vi "测试类型1can请求.vi"(3 "输入切换ID":u8, 4 "输出切换ID":u8) -> (1 "发送成功?":bool)   [LabVIEW 2010]
panel:
  in  "DataLen":i16
  in  "Data":u8[](array[numeric])
  in  "CANPort":u16
  in  "Synchronization":i32(ring)=1 items=["Synchronization"=1, "Asynchronization"=0]
  in  "WriteTimeOut":u32=5000 caption="ms"
  in  "Baudrate":u32(ring)=1000 caption="K" items=["10"=10, "20"=20, "50"=50, "100"=100, "125"=125, "250"=250, "500"=500, "800"=800, "1000"=1000]
  in  "Send_MSG":T1(array[cluster])=[{"Flags"=4, "ID(HEX)"=0, "Data "=[0, 0, 0, 0, 0, 0, 0, 0]}, {"Flags"=4, "ID(HEX)"=0, "Data "=[0, 0, 0, 0, 0, 0, 0, 1]}, {"Flags"=4, "ID(HEX)"=0, "Data "=[0, 0, 0, 0, 0, 0, 0, 2]}, {"Flags"=4, "ID(HEX)"=0, "Data "=[0, 0, 0, 0, 0, 0, 0, 3]}, {"Flags"=4, "ID(HEX)"=0, "Data "=[0, 0, 0, 0, 0, 0, 0, 4]}, {"Flags"=4, "ID(HEX)"=0, "Data "=[0, 0, 0, 0, 0, 0, 0, 5]}, {"Flags"=4, "ID(HEX)"=0, "Data "=[0, 0, 0, 0, 0, 0, 0, 6]}, {"Flags"=4, "ID(HEX)"=0, "Data "=[0, 0, 0, 0, 0, 0, 0, 7]}, {"Flags"=4, "ID(HEX)"=0, "Data "=[0, 0, 0, 0, 0, 0, 0, 8]}, {"Flags"=4, "ID(HEX)"=0, "Data "=[0, 0, 0, 0, 0, 0, 0, 9]}, {"Flags"=4, "ID(HEX)"=0, "Data "=[0, 0, 0, 0, 0, 0, 1, 0]}, {"Flags"=4, "ID(HEX)"=0, "Data "=[0, 0, 0, 0, 0, 0, 1, 1]}, {"Flags"=4, "ID(HEX)"=0, "Data "=[0, 0, 0, 0, 0, 0, 1, 2]}, {"Flags"=4, "ID(HEX)"=0, "Data "=[0, 0, 0, 0, 0, 0, 1, 3]}, {"Flags"=4, "ID(HEX)"=0, "Data "=[0, 0, 0, 0, 0, 0, 1, 4]}, {"Flags"=4, "ID(HEX)"=0, "Data "=[0, 0, 0, 0, 0, 0, 1, 5]}, {"Flags"=4, "ID(HEX)"=0, "Data "=[0, 0, 0, 0, 0, 0, 1, 6]}, {"Flags"=4, "ID(HEX)"=0, "Data "=[0, 0, 0, 0, 0, 0, 1, 7]}, {"Flags"=4, "ID(HEX)"=0, "Data "=[0, 0, 0, 0, 0, 0, 1, 8]}, {"Flags"=4, "ID(HEX)"=0, "Data "=[0, 0, 0, 0, 0, 0, 1, 9]}, {"Flags"=4, "ID(HEX)"=0, "Data "=[0, 0, 0, 0, 0, 0, 2, 0]}, {"Flags"=4, "ID(HEX)"=0, "Data "=[0, 0, 0, 0, 0, 0, 2, 1]}, {"Flags"=4, "ID(HEX)"=0, "Data "=[0, 0, 0, 0, 0, 0, 2, 2]}, {"Flags"=4, "ID(HEX)"=0, "Data "=[0, 0, 0, 0, 0, 0, 2, 3]}, {"Flags"=4, "ID(HEX)"=0, "Data "=[0, 0, 0, 0, 0, 0, 2, 4]}, {"Flags"=4, "ID(HEX)"=0, "Data "=[0, 0, 0, 0, 0, 0, 2, 5]}, {"Flags"=4, "ID(HEX)"=0, "Data "=[0, 0, 0, 0, 0, 0, 2, 6]}, {"Flags"=4, "ID(HEX)"=0, "Data "=[0, 0, 0, 0, 0, 0, 2, 7]}, {"Flags"=4, "ID(HEX)"=0, "Data "=[0, 0, 0, 0, 0, 0, 2, 8]}, {"Flags"=4, "ID(HEX)"=0, "Data "=[0, 0, 0, 0, 0, 0, 2, 9]}, {"Flags"=4, "ID(HEX)"=0, "Data "=[0, 0, 0, 0, 0, 0, 3, 0]}, {"Flags"=4, "ID(HEX)"=0, "Data "=[0, 0, 0, 0, 0, 0, 3, 1]}, {"Flags"=4, "ID(HEX)"=0, "Data "=[0, 0, 0, 0, 0, 0, 3, 2]}, {"Flags"=4, "ID(HEX)"=0, "Data "=[0, 0, 0, 0, 0, 0, 3, 3]}, {"Flags"=4, "ID(HEX)"=0, "Data "=[0, 0, 0, 0, 0, 0, 3, 4]}, {"Flags"=4, "ID(HEX)"=0, "Data "=[0, 0, 0, 0, 0, 0, 3, 5]}, {"Flags"=4, "ID(HEX)"=0, "Data "=[0, 0, 0, 0, 0, 0, 3, 6]}, {"Flags"=4, "ID(HEX)"=0, "Data "=[0, 0, 0, 0, 0, 0, 3, 7]}, {"Flags"=4, "ID(HEX)"=0, "Data "=[0, 0, 0, 0, 0, 0, 3, 8]}, {"Flags"=4, "ID(HEX)"=0, "Data "=[0, 0, 0, 0, 0, 0, 3, 9]}, {"Flags"=4, "ID(HEX)"=0, "Data "=[0, 0, 0, 0, 0, 0, 4, 0]}, {"Flags"=4, "ID(HEX)"=0, "Data "=[0, 0, 0, 0, 0, 0, 4, 1]}, {"Flags"=4, "ID(HEX)"=0, "Data "=[0, 0, 0, 0, 0, 0, 4, 2]}, {"Flags"=4, "ID(HEX)"=0, "Data "=[0, 0, 0, 0, 0, 0, 4, 3]}, {"Flags"=4, "ID(HEX)"=0, "Data "=[0, 0, 0, 0, 0, 0, 4, 4]}, {"Flags"=4, "ID(HEX)"=0, "Data "=[0, 0, 0, 0, 0, 0, 4, 5]}, {"Flags"=4, "ID(HEX)"=0, "Data "=[0, 0, 0, 0, 0, 0, 4, 6]}, {"Flags"=4, "ID(HEX)"=0, "Data "=[0, 0, 0, 0, 0, 0, 4, 7]}, {"Flags"=4, "ID(HEX)"=0, "Data "=[0, 0, 0, 0, 0, 0, 4, 8]}, {"Flags"=4, "ID(HEX)"=0, "Data "=[0, 0, 0, 0, 0, 0, 4, 9]}, {"Flags"=4, "ID(HEX)"=0, "Data "=[0, 0, 0, 0, 0, 0, 5, 0]}, {"Flags"=4, "ID(HEX)"=0, "Data "=[0, 0, 0, 0, 0, 0, 5, 1]}, {"Flags"=4, "ID(HEX)"=0, "Data "=[0, 0, 0, 0, 0, 0, 5, 2]}, {"Flags"=4, "ID(HEX)"=0, "Data "=[0, 0, 0, 0, 0, 0, 5, 3]}, {"Flags"=4, "ID(HEX)"=0, "Data "=[0, 0, 0, 0, 0, 0, 5, 4]}, {"Flags"=4, "ID(HEX)"=0, "Data "=[0, 0, 0, 0, 0, 0, 5, 5]}, {"Flags"=4, "ID(HEX)"=0, "Data "=[0, 0, 0, 0, 0, 0, 5, 6]}, {"Flags"=4, "ID(HEX)"=0, "Data "=[0, 0, 0, 0, 0, 0, 5, 7]}, {"Flags"=4, "ID(HEX)"=0, "Data "=[0, 0, 0, 0, 0, 0, 5, 8]}, {"Flags"=4, "ID(HEX)"=0, "Data "=[0, 0, 0, 0, 0, 0, 5, 9]}, {"Flags"=4, "ID(HEX)"=0, "Data "=[0, 0, 0, 0, 0, 0, 6, 0]}, {"Flags"=4, "ID(HEX)"=0, "Data "=[0, 0, 0, 0, 0, 0, 6, 1]}, {"Flags"=4, "ID(HEX)"=0, "Data "=[0, 0, 0, 0, 0, 0, 6, 2]}, {"Flags"=4, "ID(HEX)"=0, "Data "=[0, 0, 0, 0, 0, 0, 6, 3]}, {"Flags"=4, "ID(HEX)"=0, "Data "=[0, 0, 0, 0, 0, 0, 6, 4]}, {"Flags"=4, "ID(HEX)"=0, "Data "=[0, 0, 0, 0, 0, 0, 6, 5]}, {"Flags"=4, "ID(HEX)"=0, "Data "=[0, 0, 0, 0, 0, 0, 6, 6]}, {"Flags"=4, "ID(HEX)"=0, "Data "=[0, 0, 0, 0, 0, 0, 6, 7]}, {"Flags"=4, "ID(HEX)"=0, "Data "=[0, 0, 0, 0, 0, 0, 6, 8]}, {"Flags"=4, "ID(HEX)"=0, "Data "=[0, 0, 0, 0, 0, 0, 6, 9]}, {"Flags"=4, "ID(HEX)"=0, "Data "=[0, 0, 0, 0, 0, 0, 7, 0]}, {"Flags"=4, "ID(HEX)"=0, "Data "=[0, 0, 0, 0, 0, 0, 7, 1]}, {"Flags"=4, "ID(HEX)"=0, "Data "=[0, 0, 0, 0, 0, 0, 7, 2]}, {"Flags"=4, "ID(HEX)"=0, "Data "=[0, 0, 0, 0, 0, 0, 7, 3]}, {"Flags"=4, "ID(HEX)"=0, "Data "=[0, 0, 0, 0, 0, 0, 7, 4]}, {"Flags"=4, "ID(HEX)"=0, "Data "=[0, 0, 0, 0, 0, 0, 7, 5]}, {"Flags"=4, "ID(HEX)"=0, "Data "=[0, 0, 0, 0, 0, 0, 7, 6]}, {"Flags"=4, "ID(HEX)"=0, "Data "=[0, 0, 0, 0, 0, 0, 7, 7]}, {"Flags"=4, "ID(HEX)"=0, "Data "=[0, 0, 0, 0, 0, 0, 7, 8]}, {"Flags"=4, "ID(HEX)"=0, "Data "=[0, 0, 0, 0, 0, 0, 7, 9]}, {"Flags"=4, "ID(HEX)"=0, "Data "=[0, 0, 0, 0, 0, 0, 8, 0]}, {"Flags"=4, "ID(HEX)"=0, "Data "=[0, 0, 0, 0, 0, 0, 8, 1]}, {"Flags"=4, "ID(HEX)"=0, "Data "=[0, 0, 0, 0, 0, 0, 8, 2]}, {"Flags"=4, "ID(HEX)"=0, "Data "=[0, 0, 0, 0, 0, 0, 8, 3]}, {"Flags"=4, "ID(HEX)"=0, "Data "=[0, 0, 0, 0, 0, 0, 8, 4]}, {"Flags"=4, "ID(HEX)"=0, "Data "=[0, 0, 0, 0, 0, 0, 8, 5]}, {"Flags"=4, "ID(HEX)"=0, "Data "=[0, 0, 0, 0, 0, 0, 8, 6]}, {"Flags"=4, "ID(HEX)"=0, "Data "=[0, 0, 0, 0, 0, 0, 8, 7]}, {"Flags"=4, "ID(HEX)"=0, "Data "=[0, 0, 0, 0, 0, 0, 8, 8]}, {"Flags"=4, "ID(HEX)"=0, "Data "=[0, 0, 0, 0, 0, 0, 8, 9]}, {"Flags"=4, "ID(HEX)"=0, "Data "=[0, 0, 0, 0, 0, 0, 9, 0]}, {"Flags"=4, "ID(HEX)"=0, "Data "=[0, 0, 0, 0, 0, 0, 9, 1]}, {"Flags"=4, "ID(HEX)"=0, "Data "=[0, 0, 0, 0, 0, 0, 9, 2]}, {"Flags"=4, "ID(HEX)"=0, "Data "=[0, 0, 0, 0, 0, 0, 9, 3]}, {"Flags"=4, "ID(HEX)"=0, "Data "=[0, 0, 0, 0, 0, 0, 9, 4]}, {"Flags"=4, "ID(HEX)"=0, "Data "=[0, 0, 0, 0, 0, 0, 9, 5]}, {"Flags"=4, "ID(HEX)"=0, "Data "=[0, 0, 0, 0, 0, 0, 9, 6]}, {"Flags"=4, "ID(HEX)"=0, "Data "=[0, 0, 0, 0, 0, 0, 9, 7]}, {"Flags"=4, "ID(HEX)"=0, "Data "=[0, 0, 0, 0, 0, 0, 9, 8]}, {"Flags"=4, "ID(HEX)"=0, "Data "=[0, 0, 0, 0, 0, 0, 9, 9]}] {"Data" format="%x"; "Flags" items=["MSG_STD"=0, "MSG_EXT"=4]; "ID(HEX)" format="%x"}
  out "Error out":errorcluster {"code" format="%.0x"}
  in  "CANID":u32 format="%x"
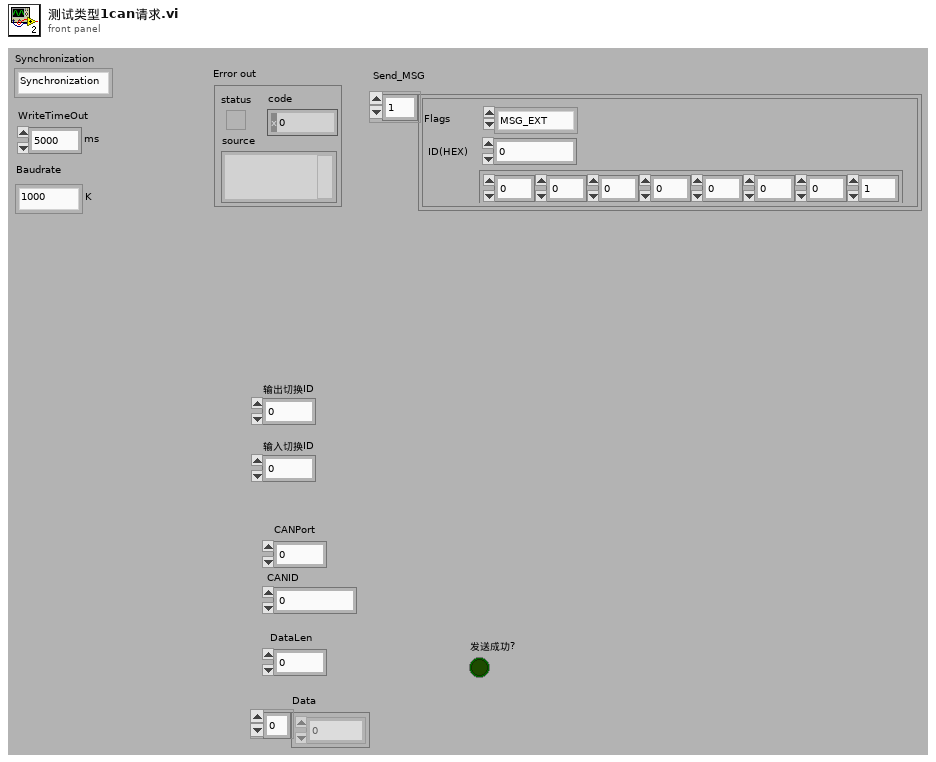
[diagram p1: front panel]
types:
  T1 = cluster{"Flags":u32, "ID(HEX)":u32, "Data ":u8[]}[]
  T2 = cluster{"Internal":u32, "InternalHigh":u32, "Offset":u32, "OffsetHigh":u32, "hEvent":u32}
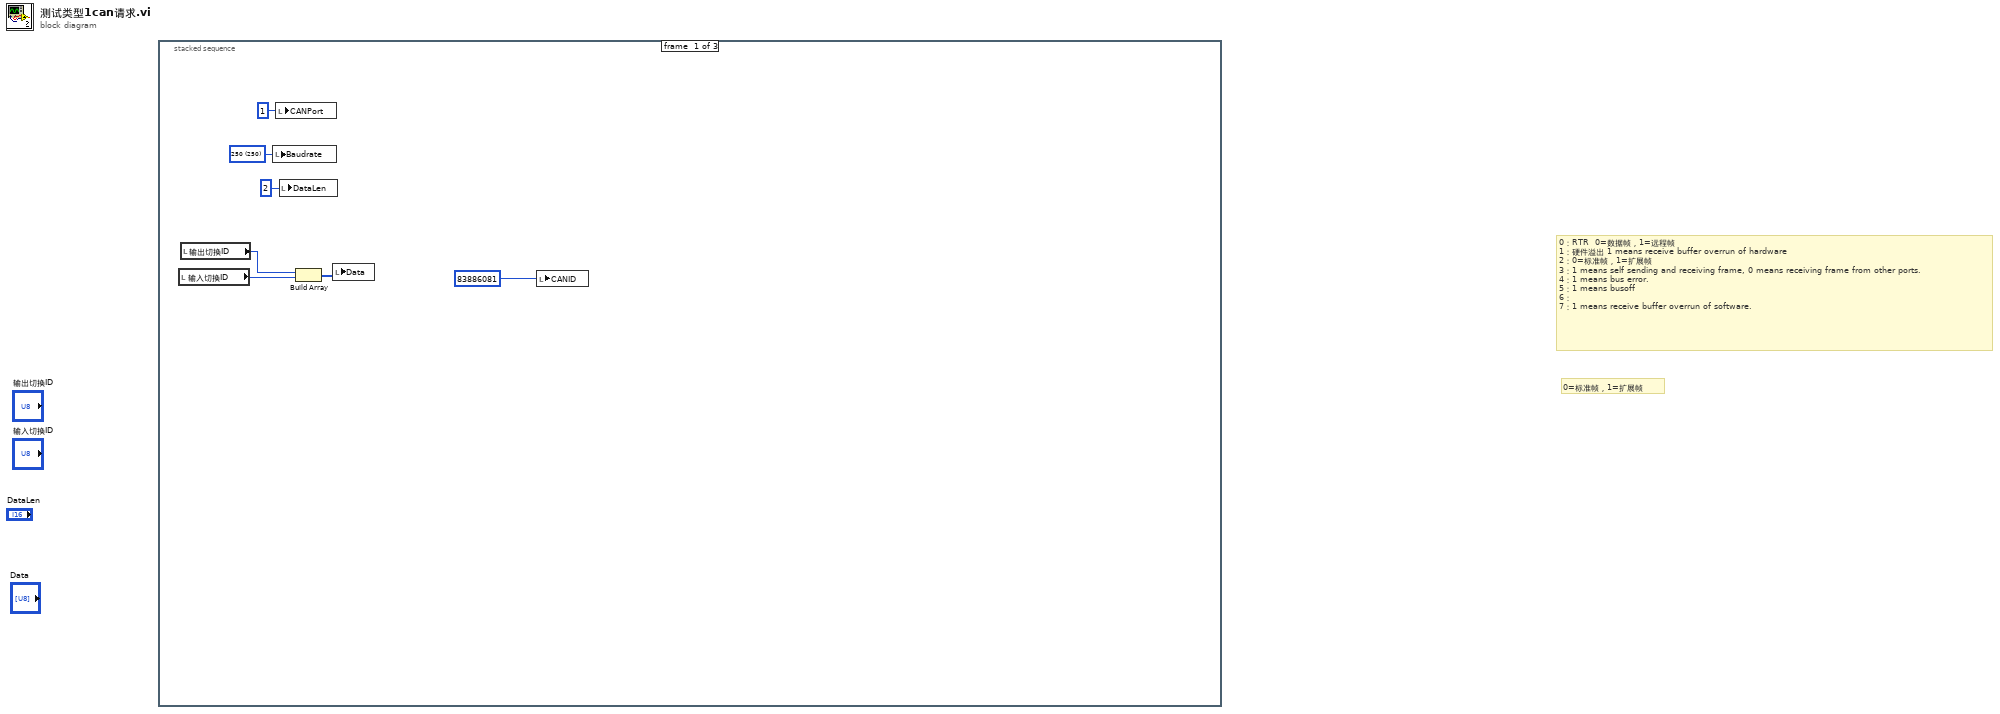
[diagram p0: block diagram]
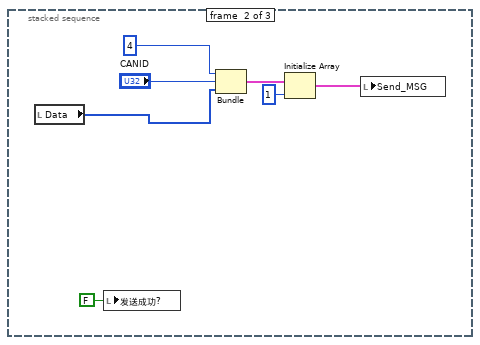
[diagram p2: hidden frame]
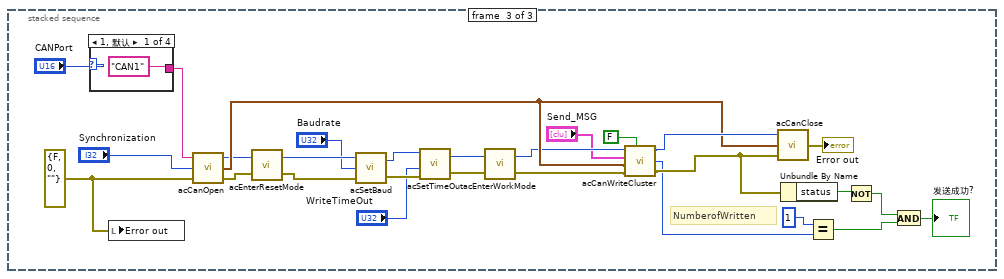
[diagram p3: hidden frame]
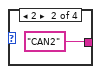
[diagram p4: hidden frame]
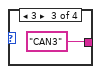
[diagram p5: hidden frame]
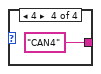
[diagram p6: hidden frame]
diagram:
  # "0=标准帧，1=扩展帧"
  # "0：RTR  0=数据帧，1=远程帧\n1：硬件溢出 1 means receive buffer overrun of hardware\n2：0=标准帧，1=扩展帧\n3：1 means self sending and receiving frame, 0 means receiving frame from other ports.\n4：1 means bus error.\n5：1 means busoff\n6：\n7：1 means receive buffer overrun of software."
  n1 = stacked-sequence {
    frame #0 {
      w7 = u32 250 items=["10"=10, "20"=20, "50"=50, "100"=100, "125"=125, "250"=250, "500"=500, "800"=800, "1000"=1000] ("Baudrate")
      n2 = local read "输入切换ID"() -> (w2:u8)
      n3 = local read "输出切换ID"() -> (w3:u8)
      n4 = local write "Baudrate"(w7) -> ()
      n5 = local write "CANPort"(u16 1 ("CANPort")) -> ()
      n6 = local write "DataLen"(i16 2 ("DataLen")) -> ()
      n7 = Build Array(w3, w2) -> (w4:u8[])
      n8 = local write "Data"(w4) -> ()
      n9 = local write "CANID"(u32 83886081 ("CANID")) -> ()
    }
    frame #1 {
      n10 = local read "Data"() -> (w8:u8[])
      n11 = local write "发送成功?"(FALSE ("发送成功?")) -> ()
      n12 = Bundle(u32 4, "CANID"="CANID", "Data"=w8) -> (w14:cluster{u32, "CANID":u32, "Data":u8[]})  [unwired: 1 in]
      n13 = Initialize Array(w14, 1 ("维数大小")) -> (w10:cluster{u32, "CANID":u32, "Data":u8[]}[])
      n14 = local write "Send_MSG"(w10) -> ()
    }
    frame #2 {
      w32 = errorcluster {"status"=FALSE, "code"=0, "source"=""} ("Error in")
      # "NumberofWritten"
      n15 = case shown="1, 默认" "CANPort" {
        tunnel: ["CAN1" "CAN2" "CAN3" "CAN4"] -> w24
        frame 1, Default {
        }
        frame 2 {
        }
        frame 3 {
        }
        frame 4 {
        }
      }
      n16 = local write "Error out"(w32) -> ()
      n17 = call "acCanOpen.vi"("Error in"=w32, "Synchronization"="Synchronization", "CANPort"=w24) -> ("Error out"=w29:errorcluster, "Overlapped"=w40:T2, "Handle"=w30:u32)
      n18 = call "acEnterResetMode.vi"("Error in"=w29, "Handle  in"=w30) -> ("Error out"=w38:errorcluster, "Handle out"=w37:u32)
      n19 = call "acSetBaud.vi"("Error in"=w38, "Baudrate"="Baudrate", "Handle  in"=w37) -> ("Error out"=w39:errorcluster, "Handle out"=w26:u32)
      n20 = call "acSetTimeOut.vi"("Error in"=w39, "WriteTimeOut"="WriteTimeOut", "Handle  in"=w26) -> ("Error out"=w33:errorcluster, "Handle out"=w34:u32)  [unwired: 1 in]
      n21 = call "acEnterWorkMode.vi"("Error in"=w33, "Handle  in"=w34) -> ("Error out"=w28:errorcluster, "Handle out"=w27:u32)
      n22 = call "acCanWriteCluster.vi"("Handle  in"=w27, "MSG"="Send_MSG", "Overlapped"=w40, "Error in"=w28, "MSG_RTR"=FALSE) -> ("Handle out"=w41:u32, "NumberOfWritten"=w15:u32, "Error out"=w42:errorcluster)
      n23 = call "acCanClose.vi"("Error in"=w42, "Overlapped"=w40, "Handle  in"=w41) -> ("Error out"=→"Error out":errorcluster)
      n24 = Unbundle By Name(w42) -> ("status"=w20:bool)
      n25 = Equal?(x=u32 1, y=w15) -> (x = y?=w18:bool)
      n26 = Not(x=w20) -> (.not. x?=w21:bool)
      n27 = And(x=w21, y=w18) -> (x .and. y?=→"发送成功?":bool)
    }
  }
